vi "PowerIn MSMT Set Reference Level.vi"(8 "error in (no error)":errorcluster, 10 "Step In":refnum<k7>, 11 "Input Power MSMT in":refnum<class "Input Power Measurement.lvclass">) -> (0 "error out":errorcluster, 2 "Step Out":refnum<k7>, 3 "Input Power MSMT out":refnum<class "Input Power Measurement.lvclass">)   [LabVIEW 2018, in "Input Power Measurement.lvlib" / "Input Power Measurement.lvclass"]
uses:
  Input Power Measurement.lvclass
  C:/P4/Sales/Semi/projects/Sequence Automation/dev/HiSi/18.0/Plugins/Measurements/Servo MSMT.lvlibp/Servo MSMT.lvclass
  Plugins/Measurement Interface.lvlibp/Measurement Interface.lvclass
  C:/P4/Sales/Semi/projects/Sequence Automation/dev/HiSi/18.0/Plugins/Measurement Interface.lvlibp/Measurement Interface.lvclass
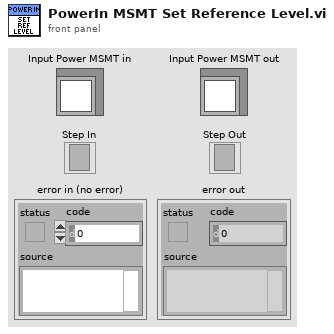
[diagram p1: front panel]
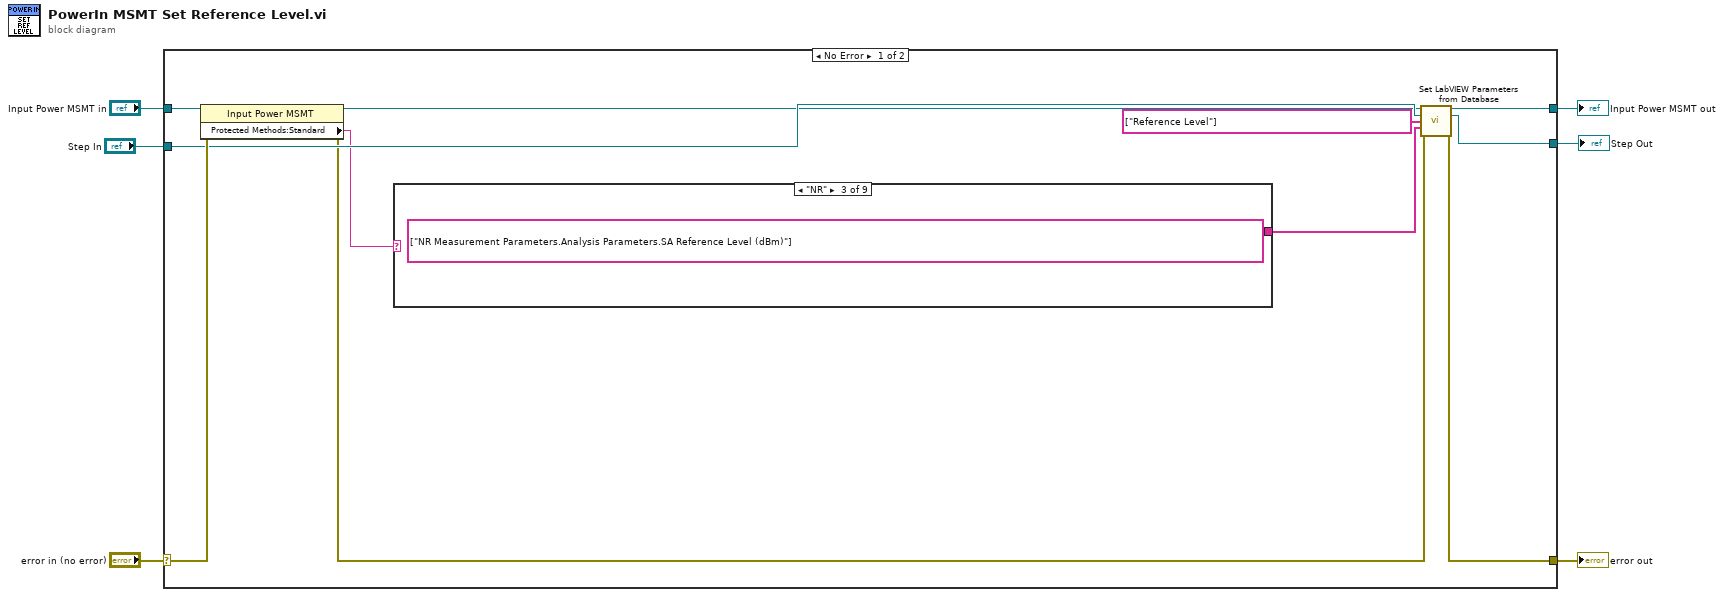
[diagram p0: block diagram]
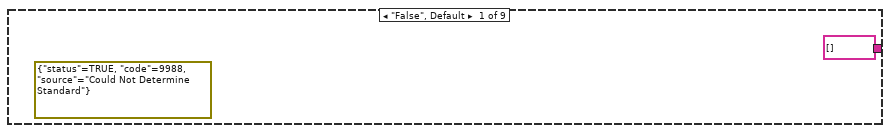
[diagram p2: hidden frame]
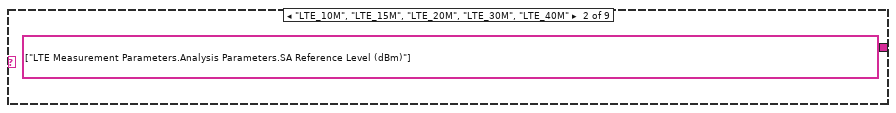
[diagram p3: hidden frame]
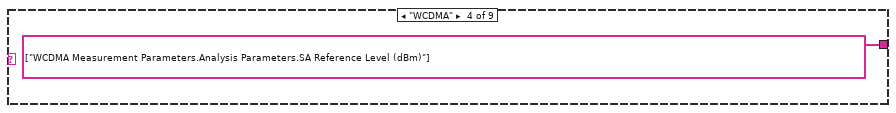
[diagram p4: hidden frame]
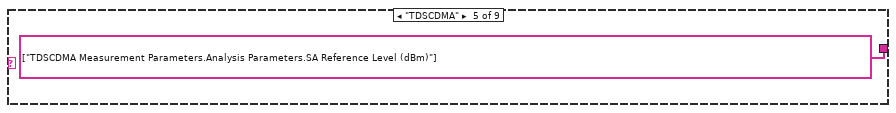
[diagram p5: hidden frame]
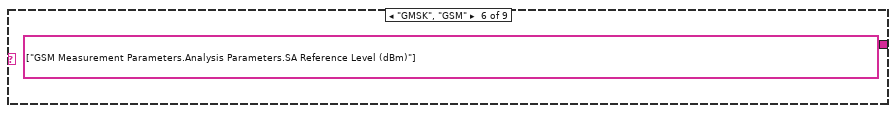
[diagram p6: hidden frame]
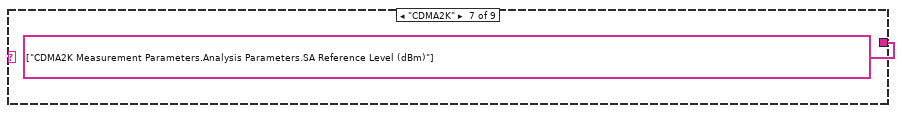
[diagram p7: hidden frame]
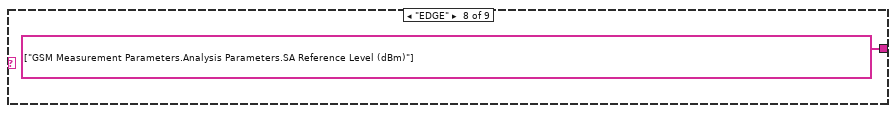
[diagram p8: hidden frame]
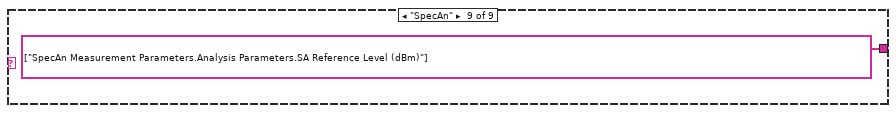
[diagram p9: hidden frame]
diagram:
  n1 = case shown="No Error" "error in (no error)" {
    selector: "error in (no error)" -> [w17 w29]
    tunnel: [w16 w29] -> w5
    tunnel: [w15 w28] -> w3
    tunnel: "Input Power MSMT in" -> [w9 w28]
    tunnel: [w12 w27] -> w2
    tunnel: "Step In" -> [w11 w27]
    frame No Error {
      n2 = property class="Input Power MSMT"(reference=w9, error in=w17) -> (reference out=w8:refnum<class "Input Power Measurement.lvclass">, error out=w10:errorcluster, "Protected Methods:Standard"=w7:string)
      n3 = case shown="\"NR\"" w7 {
        tunnel: [string[] [] string[] ["LTE Measurement Parameters.Analysis Parameters.SA Reference Level (dBm)"] string[] ["NR Measurement Parameters.Analysis Parameters.SA Reference Level (dBm)"] string[] ["WCDMA Measurement Parameters.Analysis Parameters.SA Reference Level (dBm)"] string[] ["TDSCDMA Measurement Parameters.Analysis Parameters.SA Reference Level (dBm)"] string[] ["GSM Measurement Parameters.Analysis Parameters.SA Reference Level (dBm)"] string[] ["CDMA2K Measurement Parameters.Analysis Parameters.SA Reference Level (dBm)"] string[] ["GSM Measurement Parameters.Analysis Parameters.SA Reference Level (dBm)"] string[] ["SpecAn Measurement Parameters.Analysis Parameters.SA Reference Level (dBm)"]] -> w13
        frame "False", Default {
          (unwired) errorcluster {"status"=TRUE, "code"=9988, "source"="Could Not Determine Standard"} ("error out")
        }
        frame "LTE_10M", "LTE_15M", "LTE_20M", "LTE_30M", "LTE_40M" {
        }
        frame "NR" {
        }
        frame "WCDMA" {
        }
        frame "TDSCDMA" {
        }
        frame "GMSK", "GSM" {
        }
        frame "CDMA2K" {
        }
        frame "EDGE" {
        }
        frame "SpecAn" {
        }
      }
      n4 = call "Set LabVIEW Parameters from Database.vi"("Measurement Interface in"=w8, "Step In"=w11, "Dictionary Keys"=string[] ["Reference Level"], "LabVIEW Parameter Mapping"=w13, "error in (no error)"=w10) -> ("Measurement Interface out"=w15:refnum<class "Input Power Measurement.lvclass">, "Step Out"=w12:refnum<k7>, "error out"=w16:errorcluster)  [unwired: 8 in]
    }
    frame Error {
    }
  }
  "error out" <- w5
  "Input Power MSMT out" <- w3
  "Step Out" <- w2
